vi "matlab_TI2_init.vi"(8 "error in":errorcluster) -> (0 "error out":errorcluster)   [LabVIEW 2018]
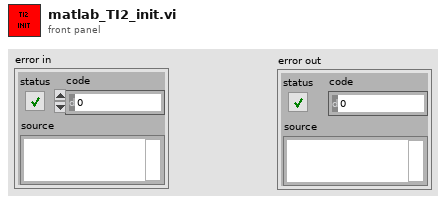
[diagram p1: front panel]
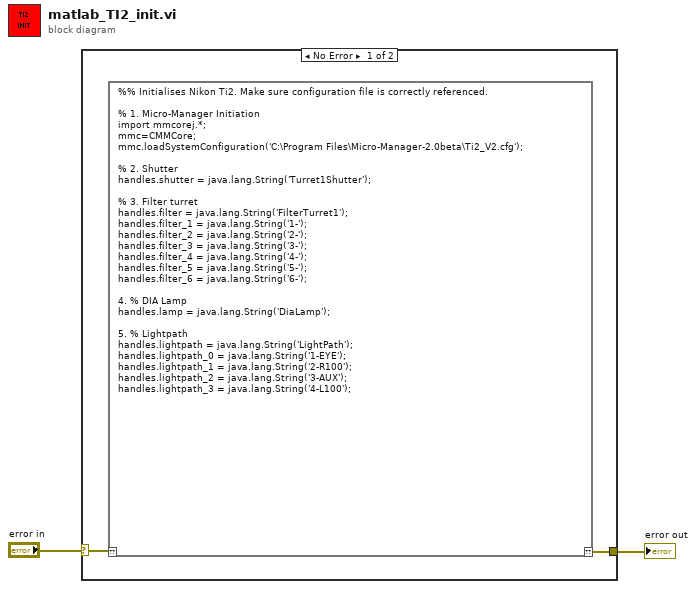
[diagram p0: block diagram]
diagram:
  n1 = case shown="No Error" "error in" {
    selector: "error in" -> [w4 w5]
    tunnel: [w3 w5] -> w1
    frame No Error {
      n2 = script code="%% Initialises Nikon Ti2. Make sure configuration file is correctly referenced.\n\n% 1. Micro-Manager Initiation\nimport mmcorej.*;\nmmc=CMMCore;\nmmc.loadSystemConfiguration('C:\\Program Files\\Micro-Manager-2.0beta\\Ti2_V2.cfg');\n\n% 2. Shutter\nhandles.shutter = java.lang.String('Turret1Shutter');\n\n% 3. Filter turret\nhandles.filter = java.lang.String('FilterTurret1');\nhandles.filter_1 = java.lang.String('1-');\nhandles.filter_2 = java.lang.String('2-');\nhandles.filter_3 = java.lang.String('3-');\nhandles.filter_4 = java.lang.String('4-');\nhandles.filter_5 = java.lang.String('5-');\nhandles.filter_6 = java.lang.String('6-');\n\n4. % DIA Lamp\nhandles.lamp = java.lang.String('DiaLamp');\n\n5. % Lightpath\nhandles.lightpath = java.lang.String('LightPath');\nhandles.lightpath_0 = java.lang.String('1-EYE');\nhandles.lightpath_1 = java.lang.String('2-R100');\nhandles.lightpath_2 = java.lang.String('3-AUX');\nhandles.lightpath_3 = java.lang.String('4-L100');"("??"=w4) -> ("??"=w3:errorcluster)
    }
    frame Error {
    }
  }
  "error out" <- w1
